vi "Write Power.AV.vi"(8 "error in":errorcluster, 10 "Power.AV":dbl, 11 "Cycler in":refnum<class "Cycler.lvclass">) -> (0 "error out":errorcluster, 3 "Cycler out":refnum<class "Cycler.lvclass">)   [LabVIEW 2023, in "Cycler.lvclass"]
uses:
  Cycler.lvclass
  Cycler.lvclass/Cycler.ctl
  <vilib>/ADAS Replay HIL/Channels/Tag Wrapper/Tag Wrapper.lvlib
  <vilib>/ADAS Replay HIL/Channels/Tag Wrapper/Polymorphic/Write Channel (Double).vi
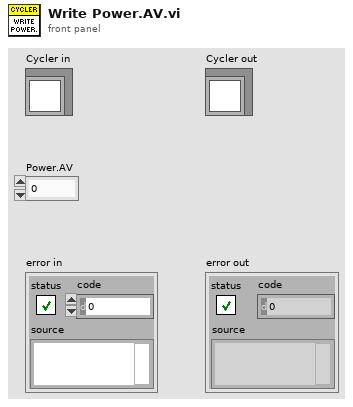
[diagram p1: front panel]
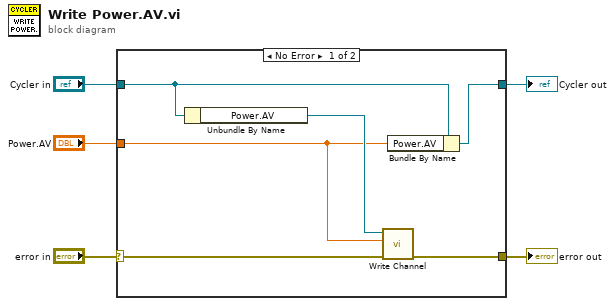
[diagram p0: block diagram]
diagram:
  n1 = case shown="No Error" "error in" {
    selector: "error in" -> [w8 w12]
    tunnel: [w9 w12] -> w4
    tunnel: [w11 w13] -> w2
    tunnel: "Cycler in" -> [w10 w13]
    tunnel: "Power.AV" -> [w6 _]
    frame No Error {
      n2 = Unbundle By Name(w10) -> ("Power.AV"=w7:refnum<k21>)
      n3 = call-poly <vilib>:"Write Channel.vi"("error in"=w8, "Value to Write"=w6, "ADAS HIL Channel in"=w7) -> ("error out"=w9:errorcluster)  [unwired: 6 in, 2 out]
      n4 = Bundle By Name(cluster=w10, "Power.AV"=w6) -> (w11:refnum<class "Cycler.lvclass">)
    }
    frame Error {
    }
  }
  "error out" <- w4
  "Cycler out" <- w2
